vi "GUI Waveform.vi"() -> ()   [LabVIEW 2020]
uses:
  Measurement/Type definitions/Measuement properties.ctl
  Measurement/Type definitions/Measurement ID.ctl
  Measurement/Type definitions/Trigger mode.ctl
  8488b85f-31b9-4e11-9177-a37569a003a1.vi
  <vilib>/Comparison/Equal/Equal Functor/Equal Functor.lvclass
panel:
  out "wave picture":picture
  in  "hide":bool
  out "waveform array storage":picture[](array[picture])=[bytes[281430], bytes[281430], bytes[281430], bytes[0], bytes[281430], bytes[281430], bytes[281430], bytes[281430], bytes[281430], bytes[281430]]
  out "Signal periods":i32[](array[numeric])
  in  "Signal label":string[](array[string])=["\n\nDigitizer 1", "\n\nDigitizer 2", "\n\nDigitizer 3", "\n\nDigitizer 4", "\n\nDigitizer 5", "\n\nDigitizer 6", "\n\nDigitizer 7", "\n\nDigitizer 8", "Digitizer 8"] caption="Signal"
  out "Waveforms":picture[][](array[picture])
  # "time (s)"
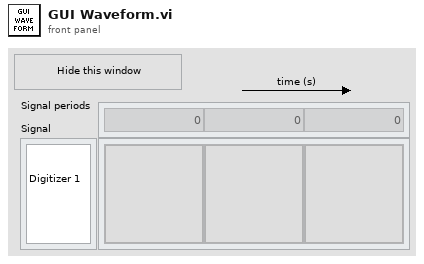
[diagram p1: front panel]
types:
  T1 = typedef "imagedata.ctl" = cluster{"image type":i32, "image depth":i32, "image":u8[], "mask":u8[], "colors":u32[], "Rectangle":cluster{"left":i16, "top":i16, "right":i16, "bottom":i16}}
  T2 = typedef "Measuement properties.ctl" = cluster{"Measurement ID":T3, "Description":string, "Switching matrix M":i32[][], "Signal frequency  (Hz)":dbl, "Maximal signal amplitude (V)":dbl, "PRs (samples)":u32, "PRe (samples)":u32, "MRs (samples)":u32, "MRe (samples)":u32, "Set PJVS frequency (Hz)":dbl, "PJVS reference voltages (1 period, V)":dbl[], "Requested PJVS frequency (Hz)":dbl, "Requiested PJVS steps":u32, "Sampling f (Hz)":dbl, "Trigger mode":T4, "Timing matrix (periods)":i32[], "Record length (multiples of M)":u32, "Calculated":cluster{"Triggers to next path (line of sequence)":u32[], "Record samples":u32, "Sample indexes of switches":u32[], "PRs (s)":dbl, "PRe (s)":dbl, "MRs (s)":dbl, "MRe (s)":dbl, "Trigger frequency  (Hz)":dbl, "Measurement druation (s)":dbl, "Samples per step":dbl, "QPMX Sequence":bool[][], "PJVS segments frequency (Hz)":dbl}, "No of required digitizers":u32, "No of required transducers":u32, "Transducer correction files":path[], "Digitizer correction file":path, "Algorithm":string, "plots_level":u32, "calc results":bool}
  T3 = typedef "Measurement ID.ctl" = enum16{"Manual setup", "1 signal, 1 ADC, 1 PJVS", "1 phase (U, I), 1 ADC, 1 PJVS", "1 phase (U, I), 2 ADC, 1 PJVS", "1 phase (U, I), 3 ADC, 1 PJVS", "3 phases (U1..3, I1..3), 3 ADC, 1 PJVS"}
  T4 = typedef "Trigger mode.ctl" = enum16{"Trigger every MX switch", "Trigger every sample"}
  T5 = enum32{"Invalid", "Standard", "Closed", "Hidden", "Minimized", "Maximized"}
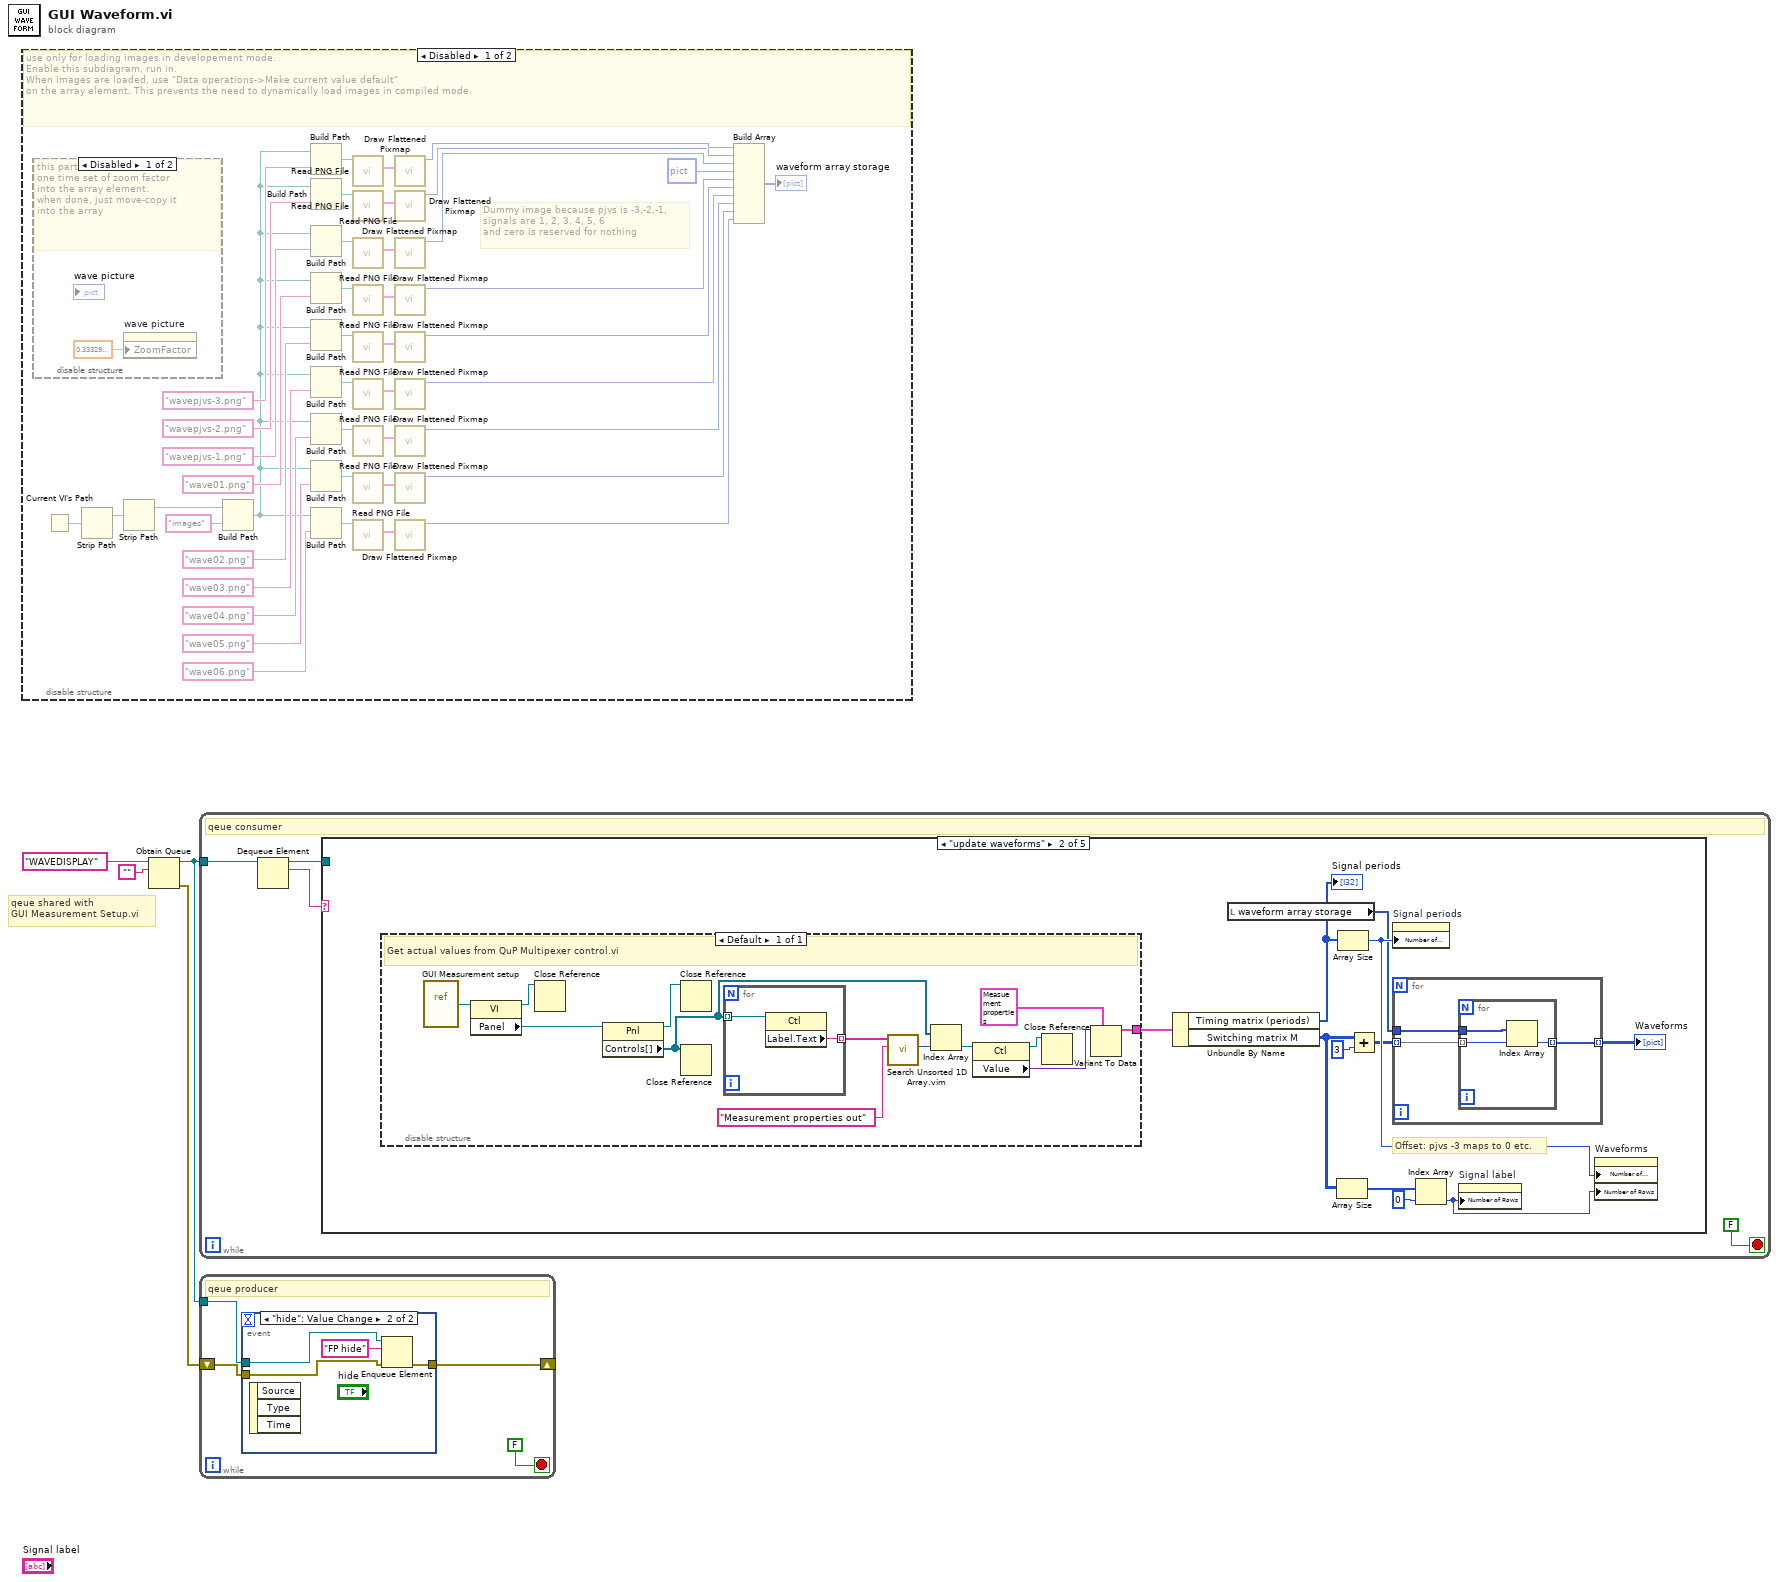
[diagram p0: block diagram]
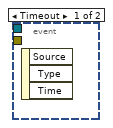
[diagram p2: hidden frame]
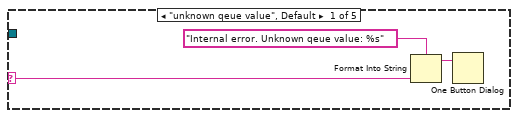
[diagram p3: hidden frame]
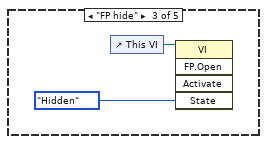
[diagram p4: hidden frame]
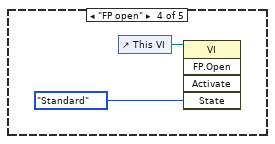
[diagram p5: hidden frame]
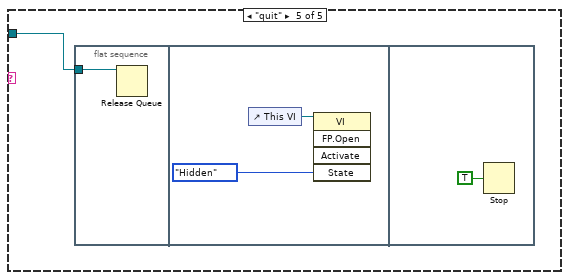
[diagram p6: hidden frame]
diagram:
  # "qeue shared with\nGUI Measurement Setup.vi"
  n1 = disable-structure shown="Disabled" {
    frame Disabled {
      # "Dummy image because pjvs is -3,-2,-1,\nsignals are 1, 2, 3, 4, 5, 6\nand zero is reserved for nothing"
      # "use only for loading images in developement mode.\nEnable this subdiagram, run in.\nWhen images are loaded, use \"Data operations->Make current value default\" \non the array element. This prevents the need to dynamically load images in compiled mode."
      n2 = disable-structure shown="Disabled" {
        frame Disabled {
          # "this part is needed for\none time set of zoom factor\ninto the array element.\nwhen done, just move-copy it \ninto the array"
          n3 = property on="wave picture" class="Pict"("ZoomFactor"=sgl 0.3333 ("Zoom Factor")) -> ()  [unwired: 2 in, 2 out]
        }
        frame Enabled {
        }
      }
      n4 = Current VI's Path() -> (path=w42:path)
      n5 = Strip Path(path=w42) -> (stripped path=w41:path)  [unwired: 1 out]
      n6 = Strip Path(path=w41) -> (stripped path=w40:path)  [unwired: 1 out]
      n7 = Build Path(base path=w40, name or relative path="images") -> (appended path=w12:path)
      n8 = Build Path(base path=w12, name or relative path="wavepjvs-3.png") -> (appended path=w37:path)
      n9 = Build Path(base path=w12, name or relative path="wavepjvs-2.png") -> (appended path=w34:path)
      n10 = Build Path(base path=w12, name or relative path="wavepjvs-1.png") -> (appended path=w32:path)
      n11 = Build Path(base path=w12, name or relative path="wave01.png") -> (appended path=w28:path)
      n12 = Build Path(base path=w12, name or relative path="wave02.png") -> (appended path=w27:path)
      n13 = Build Path(base path=w12, name or relative path="wave03.png") -> (appended path=w22:path)
      n14 = Build Path(base path=w12, name or relative path="wave04.png") -> (appended path=w13:path)
      n15 = Build Path(base path=w12, name or relative path="wave05.png") -> (appended path=w14:path)
      n16 = Build Path(base path=w12, name or relative path="wave06.png") -> (appended path=w15:path)
      n17 = call <vilib>:"Read PNG File.vi"("path to PNG file"=w37) -> ("image data"=w47:T1)  [unwired: 8 in, 2 out]
      n18 = call <vilib>:"Read PNG File.vi"("path to PNG file"=w34) -> ("image data"=w46:T1)  [unwired: 8 in, 2 out]
      n19 = call <vilib>:"Read PNG File.vi"("path to PNG file"=w32) -> ("image data"=w33:T1)  [unwired: 8 in, 2 out]
      n20 = call <vilib>:"Read PNG File.vi"("path to PNG file"=w28) -> ("image data"=w30:T1)  [unwired: 8 in, 2 out]
      n21 = call <vilib>:"Read PNG File.vi"("path to PNG file"=w27) -> ("image data"=w25:T1)  [unwired: 8 in, 2 out]
      n22 = call <vilib>:"Read PNG File.vi"("path to PNG file"=w22) -> ("image data"=w24:T1)  [unwired: 8 in, 2 out]
      n23 = call <vilib>:"Read PNG File.vi"("path to PNG file"=w13) -> ("image data"=w20:T1)  [unwired: 8 in, 2 out]
      n24 = call <vilib>:"Read PNG File.vi"("path to PNG file"=w14) -> ("image data"=w19:T1)  [unwired: 8 in, 2 out]
      n25 = call <vilib>:"Read PNG File.vi"("path to PNG file"=w15) -> ("image data"=w16:T1)  [unwired: 8 in, 2 out]
      n26 = call <vilib>:"Draw Flattened Pixmap.vi"("image data"=w47) -> ("new picture"=w45:picture)  [unwired: 8 in]
      n27 = call <vilib>:"Draw Flattened Pixmap.vi"("image data"=w46) -> ("new picture"=w44:picture)  [unwired: 8 in]
      n28 = call <vilib>:"Draw Flattened Pixmap.vi"("image data"=w33) -> ("new picture"=w31:picture)  [unwired: 8 in]
      n29 = call <vilib>:"Draw Flattened Pixmap.vi"("image data"=w30) -> ("new picture"=w11:picture)  [unwired: 8 in]
      n30 = call <vilib>:"Draw Flattened Pixmap.vi"("image data"=w25) -> ("new picture"=w5:picture)  [unwired: 8 in]
      n31 = call <vilib>:"Draw Flattened Pixmap.vi"("image data"=w24) -> ("new picture"=w10:picture)  [unwired: 8 in]
      n32 = call <vilib>:"Draw Flattened Pixmap.vi"("image data"=w20) -> ("new picture"=w9:picture)  [unwired: 8 in]
      n33 = call <vilib>:"Draw Flattened Pixmap.vi"("image data"=w19) -> ("new picture"=w8:picture)  [unwired: 8 in]
      n34 = call <vilib>:"Draw Flattened Pixmap.vi"("image data"=w16) -> ("new picture"=w7:picture)  [unwired: 8 in]
      n35 = Build Array(w45, w44, w31, picture data[5B] ("element"), w11, w5, w10, w9, w8, w7) -> (→"waveform array storage":picture[])
    }
    frame Enabled {
    }
  }
  n36 = Obtain Queue(name (unnamed)="WAVEDISPLAY", element data type="" ("data (can be any type)")) -> (queue out=w1:refnum<queue>, error out=w2:errorcluster)  [unwired: 3 in, 1 out]
  n37 = while {
    tunnel: w1 -> [w51]
    stop <- FALSE stop-if-true
    # "qeue consumer"
    n38 = Dequeue Element(queue=w51) -> (queue out=w49:refnum<queue>, element=w50:string)  [unwired: 2 in, 2 out]
    n39 = case shown="\"update waveforms\"" w50 {
      selector: w50 -> [w53 _ _ _ _]
      tunnel: w49 -> [_ _ _ _ w92]
      frame "unknown qeue value", Default {
        n40 = Format Into String(format string="Internal error. Unknown qeue value: %s", w53) -> (resulting string=w55:string)  [unwired: 2 in, 1 out]
        n41 = One Button Dialog(message=w55) -> ()  [unwired: 1 in, 1 out]
      }
      frame "update waveforms" {
        # "Offset: pjvs -3 maps to 0 etc."
        n42 = disable-structure shown="Default" {
          disable-tunnel: [w77] -> w56
          frame Enabled {
            # "Get actual values from QuP Multipexer control.vi"
            n43 = vi-ref "GUI Measurement setup.vi"() -> (w76:refnum<vi>)
            n44 = property class="VI"(reference=w76) -> (reference out=w75:refnum<vi>, "Panel"=w85:refnum<vi>)  [unwired: 1 in, 1 out]
            n45 = Close Reference(reference=w75) -> ()  [unwired: 1 in, 1 out]
            n46 = property class="Pnl"(reference=w85) -> (reference out=w78:refnum<vi>, "Controls[]"=w79:refnum<vi>[])  [unwired: 1 in, 1 out]
            n47 = Close Reference(reference=w78) -> ()  [unwired: 1 in, 1 out]
            n48 = Close Reference(reference=w79) -> ()  [unwired: 1 in, 1 out]
            n49 = for {
              tunnel: w79 -> [w87] mode=indexing
              tunnel: [w86] -> w80 mode=indexing
              n50 = property class="Ctl"(reference=w87) -> ("Label.Text"=w86:string)  [unwired: 1 in, 2 out]
            }
            n51 = call "Search Unsorted 1D Array.vim"("element"="Measurement properties out" ("Label.Text"), "unsorted 1D array"=w80) -> ("index of element"=w82:i32)  [unwired: 9 in]
            n52 = Index Array(array=w79, index=w82) -> (element=w83:refnum<vi>)
            n53 = property class="Ctl"(reference=w83) -> (reference out=w74:refnum<vi>, "Value"=w84:variant)  [unwired: 1 in, 1 out]
            n54 = Close Reference(reference=w74) -> ()  [unwired: 1 in, 1 out]
            n55 = Variant To Data(type=T2 {"Measurement ID"=enum."1 signal, 1 ADC, 1 PJVS", "Description"="3 phase, 3 ADC, 1 PJVS", "Switching matrix M"=[[1, -1, 2], [-2, 3, 4]], "Signal frequency  (Hz)"=50.0, "Maximal signal amplitude (V)"=0.0, "PRs (samples)"=0, "PRe (samples)"=0, "MRs (samples)"=0, "MRe (samples)"=0, "Set PJVS frequency (Hz)"=50.0, "PJVS reference voltages (1 period, V)"=[], "Requested PJVS frequency (Hz)"=50.0, "Requiested PJVS steps"=10, "Sampling f (Hz)"=7000.0, "Trigger mode"=enum."Trigger every MX switch", "Timing matrix (periods)"=[1, 1, 3], "Record length (multiples of M)"=1, "Calculated"={"Triggers to next path (line of sequence)"=[], "Record samples"=0, "Sample indexes of switches"=[], "PRs (s)"=0.0, "PRe (s)"=0.0, "MRs (s)"=0.0, "MRe (s)"=0.0, "Trigger frequency  (Hz)"=50.0, "Measurement druation (s)"=0.0, "Samples per step"=0.0, "QPMX Sequence"=[], "PJVS segments frequency (Hz)"=50.0}, "No of required digitizers"=0, "No of required transducers"=0, "Transducer correction files"=[], "Digitizer correction file"=path "", "Algorithm"="TWM-PWRFFT", "plots_level"=1, "calc results"=FALSE} ("Measurement properties"), Variant=w84) -> (data=w77:T2)  [unwired: 1 in, 1 out]
          }
        }
        n56 = Unbundle By Name(w56) -> ("Timing matrix (periods)"=w62:i32[], "Switching matrix M"=w64:i32[][])
        "Signal periods" <- w62
        n57 = local read "waveform array storage"() -> (w60:picture[])
        n58 = Array Size(array=w64) -> (size(s)=w65:i32[])
        n59 = Array Size(array=w62) -> (size(s)=w63:i32)
        n60 = Add(x=w64, y=u32 3 ("Number of Columns")) -> (x+y=w61:u32[][])
        n61 = property on="Signal periods" class="Arr (strict)"("Number of Columns"=w63) -> ()  [unwired: 2 in, 2 out]
        n62 = for {
          tunnel: w61 -> [w68] mode=indexing
          tunnel: w60 -> [w69]
          tunnel: [w67] -> w59 mode=indexing
          n63 = for {
            tunnel: w69 -> [w72]
            tunnel: w68 -> [w71] mode=indexing
            tunnel: [w70] -> w67 mode=indexing
            n64 = Index Array(array=w72, index=w71) -> (element=w70:picture)
          }
        }
        "Waveforms" <- w59
        n65 = Index Array(array=w65, index=0) -> (element=w66:i32)
        n66 = property on="Signal label" class="Arr (strict)"("Number of Rows"=w66) -> ()  [unwired: 2 in, 2 out]
        n67 = property on="Waveforms" class="Arr (strict)"("Number of Columns"=w63, "Number of Rows"=w66) -> ()  [unwired: 2 in, 2 out]
      }
      frame "FP hide" {
        n68 = control-ref of="This VI"() -> (w88:refnum<vi>)
        n69 = invoke class="VI" method="FP.Open"(reference=w88, "State"=T5."Hidden") -> ()  [unwired: 3 in, 5 out]
      }
      frame "FP open" {
        n70 = control-ref of="This VI"() -> (w90:refnum<vi>)
        n71 = invoke class="VI" method="FP.Open"(reference=w90, "State"=T5."Standard") -> ()  [unwired: 3 in, 5 out]
      }
      frame "quit" {
        n72 = flat-sequence {
          tunnel: w92 -> [w93]
          frame #0 {
            n73 = Release Queue(queue=w93) -> ()  [unwired: 2 in, 3 out]
          }
          frame #1 {
            n74 = control-ref of="This VI"() -> (w94:refnum<vi>)
            n75 = invoke class="VI" method="FP.Open"(reference=w94, "State"=T5."Hidden") -> ()  [unwired: 3 in, 5 out]
          }
          frame #2 {
            n76 = Stop(stop? (T)=TRUE) -> ()
          }
        }
      }
    }
  }
  n77 = while {
    shift-right: [w99] -> _
    shift-left: w2 -> [w100]
    tunnel: w1 -> [w98]
    stop <- FALSE stop-if-true
    # "qeue producer"
    n78 = event shown="[1] \"hide\": Value Change" {
      selector: _ -> [_ _]
      dyn-events: _ -> [_ _]
      timeout: _ -> [_ _]
      tunnel: w100 -> [_ w103]
      tunnel: [_ w102] -> w99
      tunnel: w98 -> [_ w101]
      event Timeout {
        n79 = event-data() -> ()  [unwired: 1 in, 3 out]
      }
      event "hide": Value Change {
        n80 = event-data() -> ()  [unwired: 1 in, 3 out]
        n81 = Enqueue Element(queue=w101, element="FP hide", error in (no error)=w103) -> (error out=w102:errorcluster)  [unwired: 1 in, 2 out]
      }
    }
  }
